vi "SingleControllerTwoStages.vi"() -> ()   [LabVIEW 2012]
uses:
  Madlib.dll
panel:
  in  "Theta y":dbl min=0.0 max=200.0 step=1.0 format="%.3f"
  out "Device 2 Theta y":dbl(graph)
  out "Device 2 Theta x":dbl(graph)
  in  "Theta x":dbl min=0.0 max=200.0 step=1.0 format="%.3f"
  in  "Theta y":dbl min=0.0 max=200.0 step=1.0 format="%.3f"
  out "Device 1 Theta y":dbl(graph)
  in  "?":dbl min=0.0 max=200.0 step=1.0 format="%.3f"
  out "Device 1 Theta x":dbl(graph)
  in  "?":bool
  # "Device 1"
  # "Device 2"
  # "Theta x"
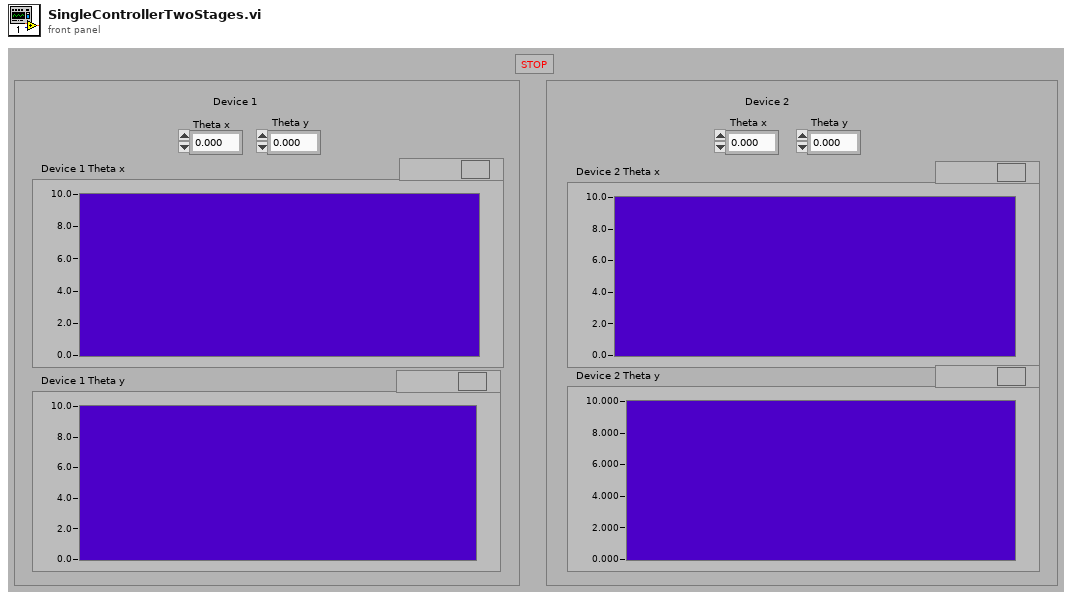
[diagram p1: front panel]
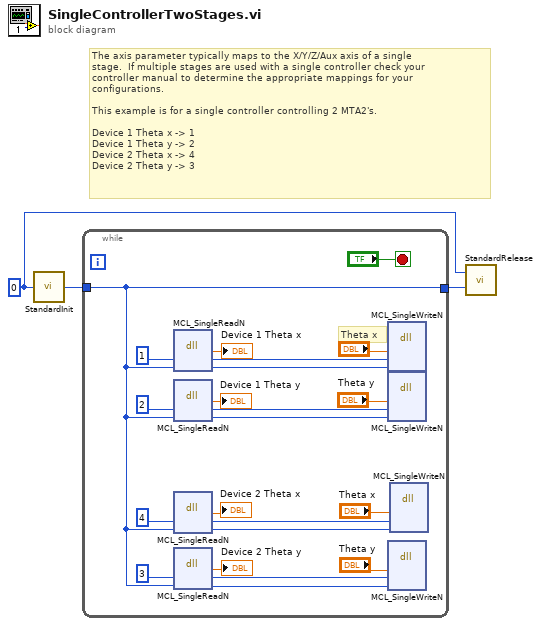
[diagram p0: block diagram]
diagram:
  w1 = 0
  # "The axis parameter typically maps to the X/Y/Z/Aux axis of a single\nstage.  If multiple stages are used with a single controller check your\ncontroller manual to determine the appropriate mappings for your\nconfigurations.  \n\nThis example is for a single controller controlling 2 MTA2's.  \n\nDevice 1 Theta x -> 1\nDevice 1 Theta y -> 2\nDevice 2 Theta x -> 4\nDevice 2 Theta y -> 3"
  n1 = call "StandardInit.vi"("Incoming Handle"=w1) -> ("Outgoing Handle"=w3:i32)
  n2 = while {
    tunnel: w3 -> [w5]
    tunnel: [w5] -> w2
    stop <- "?" stop-if-true
    # "Theta x"
    n3 = dll-call lib="C:/Users/Labview/Desktop/SRR/Madlib_x64/Labview Examples/MADLib.dll" fn="MCL_SingleReadN"("axis"=u16 1, "handle"=w5) -> (→"Device 1 Theta x":dbl, "axis"=w12:u32, "handle"=w24:i32)  [unwired: 3 in, 2 out]
    n4 = dll-call lib="C:/Users/Labview/Desktop/SRR/Madlib_x64/Labview Examples/MADLib.dll" fn="MCL_SingleReadN"("axis"=u16 2, "handle"=w5) -> (→"Device 1 Theta y":dbl, "axis"=w4:u32, "handle"=w23:i32)  [unwired: 3 in, 2 out]
    n5 = dll-call lib="C:/Users/Labview/Desktop/SRR/Madlib_x64/Labview Examples/MADLib.dll" fn="MCL_SingleReadN"("axis"=4, "handle"=w5) -> (→"Device 2 Theta x":dbl, "axis"=w11:u32, "handle"=w22:i32)  [unwired: 3 in, 2 out]
    n6 = dll-call lib="C:/Users/Labview/Desktop/SRR/Madlib_x64/Labview Examples/MADLib.dll" fn="MCL_SingleReadN"("axis"=3, "handle"=w5) -> (→"Device 2 Theta y":dbl, "axis"=w10:u32, "handle"=w21:i32)  [unwired: 3 in, 2 out]
    n7 = dll-call lib="C:/Users/Labview/Desktop/SRR/Madlib_x64/Labview Examples/MADLib.dll" fn="MCL_SingleWriteN"("position"="?", "axis"=w12, "handle"=w24) -> ()  [unwired: 7 in, 2 out]
    n8 = dll-call lib="C:/Users/Labview/Desktop/SRR/Madlib_x64/Labview Examples/MADLib.dll" fn="MCL_SingleWriteN"("position"="Theta y", "axis"=w4, "handle"=w23) -> ()  [unwired: 7 in, 2 out]
    n9 = dll-call lib="C:/Users/Labview/Desktop/SRR/Madlib_x64/Labview Examples/MADLib.dll" fn="MCL_SingleWriteN"("position"="Theta y", "axis"=w10, "handle"=w21) -> ()  [unwired: 7 in, 2 out]
    n10 = dll-call lib="C:/Users/Labview/Desktop/SRR/Madlib_x64/Labview Examples/MADLib.dll" fn="MCL_SingleWriteN"("position"="Theta x", "axis"=w11, "handle"=w22) -> ()  [unwired: 7 in, 2 out]
  }
  n11 = call "StandardRelease.vi"("Outgoing Handle"=w2, "Incoming Handle"=w1) -> ()  [unwired: 1 in]
